vi "DAQmxAI Test.vi"   [LabVIEW 2020, in "VolatusScratch.lvlib"]
uses:
  VolatusScratch.lvlib
  Volatus/Volatus Core/Volatus Core.lvclass
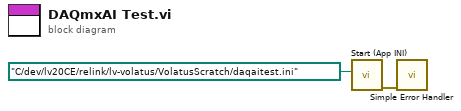
[diagram p0: block diagram]
diagram:
  n1 = call "Start (App INI).vi"("INI Path (Default)"=path "C:/dev/lv20CE/relink/lv-volatus/VolatusScratch/daqaitest.ini") -> ("error out"=w1:errorcluster)  [unwired: 9 in, 1 out]
  n2 = call <vilib>:"Simple Error Handler.vi"("error in (no error)"=w1) -> ()  [unwired: 4 in, 5 out]
